vi "Queues_global.vi"() -> ()   [LabVIEW 2019]
panel:
  out "MFL Queue":refnum<queue>
  out "Recondense Queue":refnum<queue> caption="5T Queue"
  out "SMI921 Queue":refnum<queue>
  out "Kelvinox Queue":refnum<queue>
  out "zurich_lock_in-1 Open Queue":refnum<queue>
  out "P9P14 Temp Queue":refnum<queue>
  out "TMC Queue":refnum<queue>
  out "K2182A":refnum<queue>
  out "P9P14 Queue":refnum<queue>
  out "LIA7230-3":refnum<queue>
  out "LIA7230-2":refnum<queue>
  out "LIA7230":refnum<queue>
  out "ITC503 Queue":refnum<queue>
  out "LS370 read only Queue":refnum<queue>
  out "LS372  read only Queue":refnum<queue>
  out "15T Queue":refnum<queue> caption="5T Queue"
  out "AH2700 Queue":refnum<queue> caption="Mischer Levelmeter N"
  out "AH2500 Queue":refnum<queue> caption="Mischer Levelmeter N"
  out "AMI Queue":refnum<queue> caption="Mischer Levelmeter N"
  out "Picowatt AVS47 Queue":refnum<queue> caption="Mischer Levelmeter N"
  out "PE7265 Queue":refnum<queue> caption="Mischer Levelmeter N"
  out "VCM Queue":refnum<queue> caption="Mischer Levelmeter N"
  out "Mischer Levelmeter N":refnum<queue>
  out "5T Queue":refnum<queue>
  out "K6221":refnum<queue>
  out "20T-Dewar":refnum<queue>
  out "SR830-3":refnum<queue>
  out "SR830-2":refnum<queue>
  out "ILM":refnum<queue>
  out "SR830":refnum<queue>
  out "16 T Queue":refnum<queue>
  out "VTI Queue":refnum<queue>
  out "LS372 Queue":refnum<queue>
  out "LS370 Queue":refnum<queue>
  out "JT Queue":refnum<queue>
  out "20TVTI Queue":refnum<queue>
  out "20 T Queue":refnum<queue>
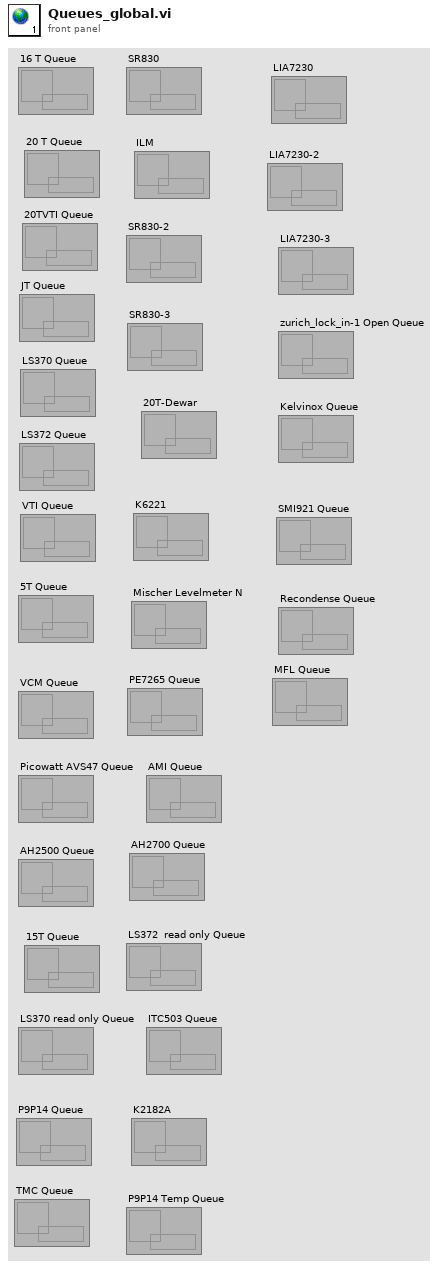
[diagram p1: front panel]
diagram:
